vi "0xFA_Program_reset.vi"(8 "error in":errorcluster, 11 "ParamIn":T1={"ReadIntParam"=TRUE, "ReadDescrParam"=FALSE, "ReadFloatParam"=TRUE, "debug"=FALSE, "ReadJSON"=TRUE, "IP_address"="192.168.1.216", "N_attempts"=3, "type_con"=enum."TCP", "MB_address"=1, "VISA"="COM1", "connection ID"=refnum, "nameDevices"="", "timeout"=0, "port"=0, "type_version"="0F0C0001", "baud_rate"=115200, "VersionControl"=TRUE, "TCP_conn"=TRUE, "WindowSize"=700}) -> (0 "error out":errorcluster, 3 "ParamOut":T1={"ReadIntParam"=TRUE, "ReadDescrParam"=FALSE, "ReadFloatParam"=TRUE, "debug"=FALSE, "ReadJSON"=TRUE, "IP_address"="192.168.1.216", "N_attempts"=3, "type_con"=enum."TCP", "MB_address"=1, "VISA"="COM1", "connection ID"=refnum, "nameDevices"="", "timeout"=0, "port"=0, "type_version"="0F0C0001", "baud_rate"=115200, "VersionControl"=TRUE, "TCP_conn"=TRUE, "WindowSize"=700})   [LabVIEW 2017, in "LV_Unicorn.lvlib"]
uses:
  LV_Unicorn.lvlib
  Control/unicorn_conn.ctl
panel:
  out "Ответ":string
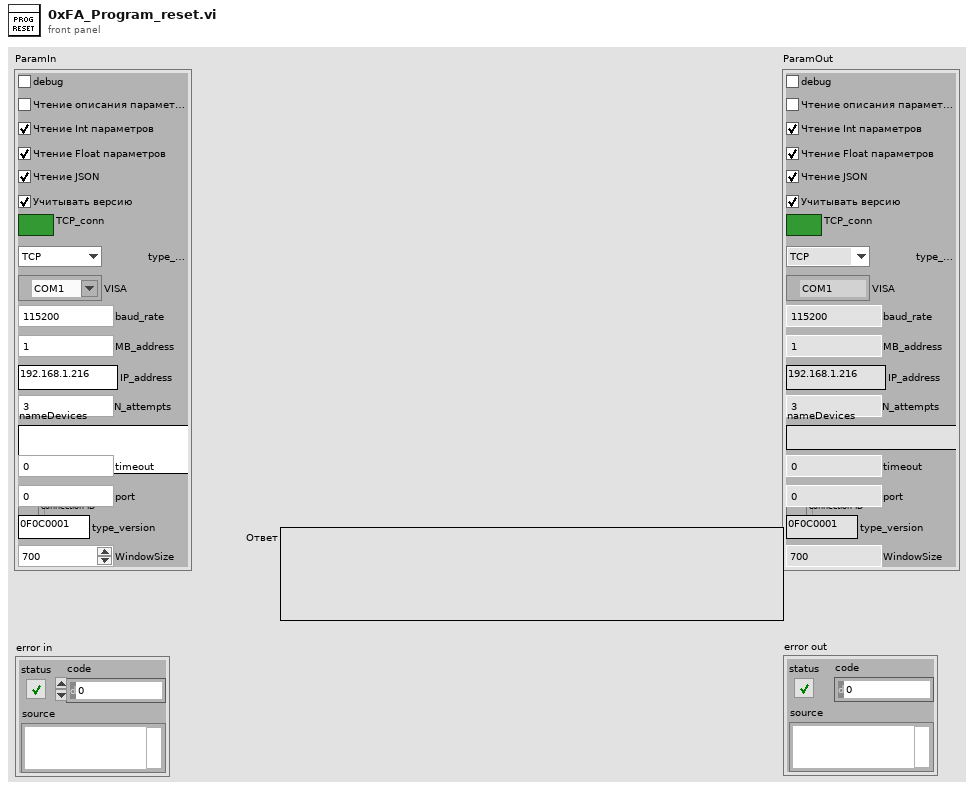
[diagram p1: front panel]
types:
  T1 = typedef "LV_Unicorn.lvlib/unicorn_conn.ctl" = cluster{"ReadIntParam":bool, "ReadDescrParam":bool, "ReadFloatParam":bool, "debug":bool, "ReadJSON":bool, "IP_address":string, "N_attempts":i32, "type_con":enum16{"Serial", "TCP"}, "MB_address":i32, "VISA":refnum<visa-resource-name>, "connection ID":refnum<k5>, "nameDevices":string, "timeout":i32, "port":u16, "type_version":string, "baud_rate":u32, "VersionControl":bool, "TCP_conn":bool, "WindowSize":i32}
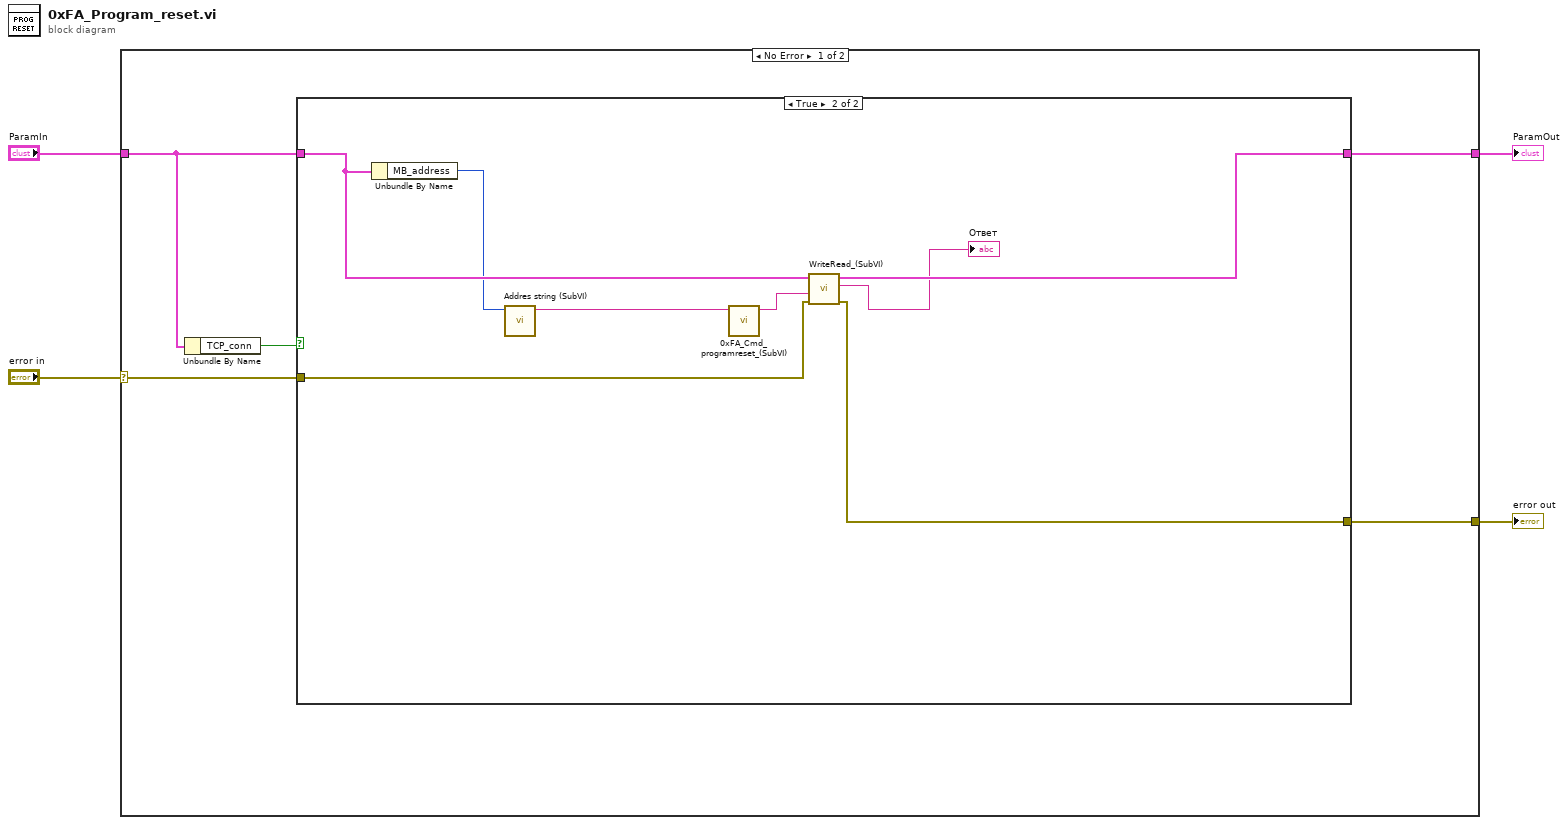
[diagram p0: block diagram]
diagram:
  n1 = case shown="No Error" "error in" {
    selector: "error in" -> [w7 w21]
    tunnel: "ParamIn" -> [w6 w20]
    tunnel: [w9 w20] -> w4
    tunnel: [w8 w21] -> w3
    frame No Error {
      n2 = Unbundle By Name(w6) -> ("TCP_conn"=w5:bool)
      n3 = case shown="True" w5 {
        tunnel: w6 -> [w10 w19]
        tunnel: [w10 w16] -> w9
        tunnel: [w11 w15] -> w8
        tunnel: w7 -> [w11 w14]
        frame False {
        }
        frame True {
          n4 = Unbundle By Name(w19) -> ("MB_address"=w17:i32)
          n5 = call "Addres string (SubVI).vi"("Адрес"=w17) -> ("String"=w18:string)  [unwired: 10 in]
          n6 = call "0xFA_Cmd_programreset_(SubVI).vi"("String in"=w18) -> ("String out"=w12:string)  [unwired: 10 in]
          n7 = call "WriteRead_(SubVI).vi"("error in"=w14, "Запрос"=w12, "ParamIn"=w19) -> ("error out"=w15:errorcluster, "Ответ"=→"Ответ":string, "ParamOut"=w16:T1)  [unwired: 4 in, 2 out]
        }
      }
    }
    frame Error {
    }
  }
  "error out" <- w3
  "ParamOut" <- w4
